vi "Array of Clusters to VMap__ogtk.vi"(8 "error in":errorcluster, 11 "Array of Clusters (key-value)":variant) -> (0 "error out":errorcluster, 3 "Map":variant)   [LabVIEW 2023, in "openg_variant.lvlib"]
uses:
  openg_variant.lvlib
panel:
  # "EXPERIMENTAL"
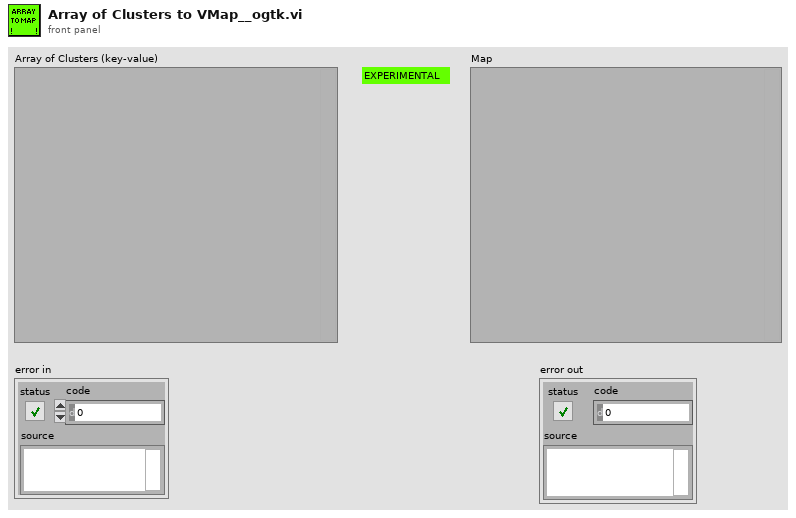
[diagram p1: front panel]
types:
  T1 = typedef "openg_variant.lvlib/Type Descriptor__ogtk.ctl" = i16[]
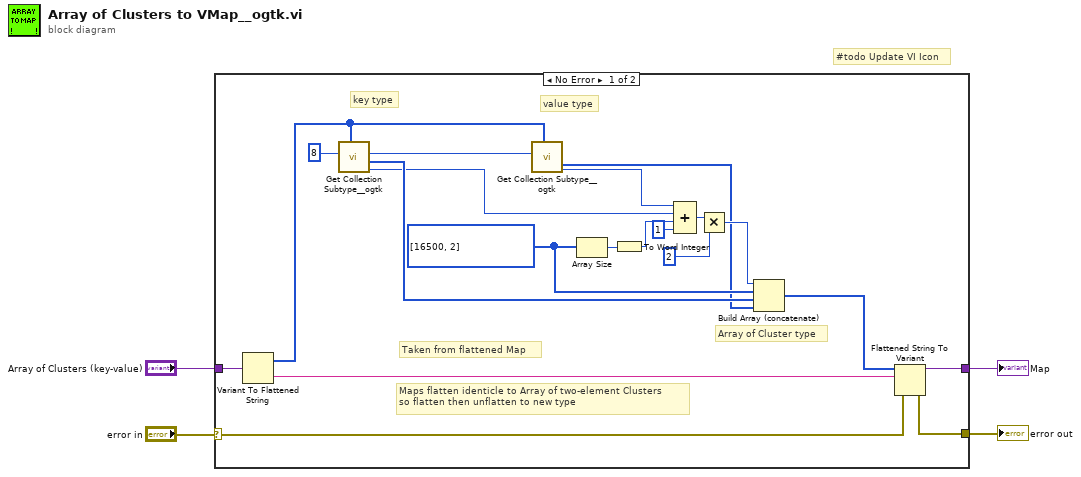
[diagram p0: block diagram]
diagram:
  # "#todo Update VI Icon"
  n1 = case shown="No Error" "error in" {
    selector: "error in" -> [w22 w25]
    tunnel: [w24 _] -> w4
    tunnel: "Array of Clusters (key-value)" -> [w23 _]
    tunnel: [w21 w25] -> w1
    frame No Error {
      w15 = i16[] [16500, 2] ("type string 7")
      # "Taken from flattened Map"
      # "Maps flatten identicle to Array of two-element Clusters\nso flatten then unflatten to new type"
      # "value type"
      # "key type"
      # "Array of Cluster type"
      n2 = Variant To Flattened String(Variant=w23) -> (data string=w17:string, 1:w5:i16[])
      n3 = call "Get Collection Subtype__ogtk.vi"("Type Descriptor"=w5, "Offset In"=i16 8 ("index")) -> ("Size"=w9:i16, "subtype"=w16:T1, "Offset out"=w8:i16)  [unwired: 7 in]
      n4 = call "Get Collection Subtype__ogtk.vi"("Type Descriptor"=w5, "Offset In"=w8) -> ("Size"=w6:i16, "subtype"=w7:T1)  [unwired: 7 in, 1 out]
      n5 = Array Size(array=w15) -> (size(s)=w14:i32)
      n6 = To Word Integer(number=w14) -> (16bit integer=w12:i16)
      n7 = Compound Arithmetic op=ADD(w6, w9, w12, i16 1 ("value")) -> (w13:i16)
      n8 = Multiply(x=w13, y=i16 2) -> (x*y=w19:i16)
      n9 = Build Array (concatenate)(w19, w15, w16, w7) -> (w18:T1)
      n10 = Flattened String To Variant(4:w22, 6:w17, 7:w18) -> (0:w21:errorcluster, 3:w24:variant)
    }
    frame Error {
    }
  }
  "Map" <- w4
  "error out" <- w1
